vi "Grid_GetAttributes.vi"(0 "reference in":refnum<class "Grid.lvclass">, 5 "error in (no error)":errorcluster) -> (14 "reference out":refnum<class "Grid.lvclass">, 16 "Attributes":T1 {"gridY" format="%.2f"; "gridX" format="%.2f"}, 17 "Attributes locked?":bool, 19 "error out":errorcluster)   [LabVIEW 2012, in "Grid.lvclass"]
doc: "Returns the attributes of a Grid or subclass object.\n\nIf the object is currently locked for modification, 'Attibutes locked?' will return TRUE.\n\n[GOOP 2.0.15]"
uses:
  <resource>/Framework/Providers/Open_GDS/UML/Grid_class/Grid.lvclass
  <resource>/Framework/Providers/Open_GDS/UML/Grid_class/protected/ObjectAttributes.ctl
  <vilib>/addons/_goop3.llb/3GOOPStates.ctl
  <resource>/Framework/Providers/Open_GDS/UML/Grid_class/Grid.lvclass/Grid.ctl
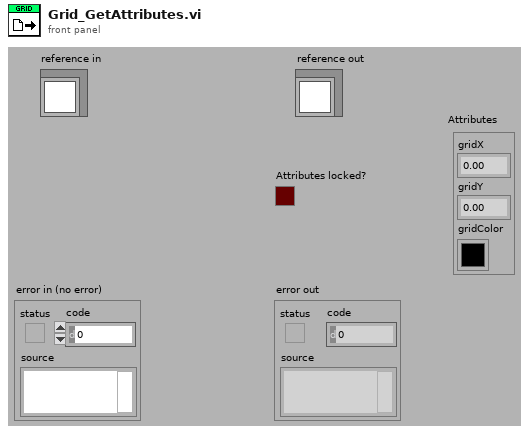
[diagram p1: front panel]
types:
  T1 = typedef "Grid.lvclass/ObjectAttributes.ctl" = cluster{"gridX":dbl, "gridY":dbl, "gridColor":u32}
  T2 = typedef "3GOOPStates.ctl" = enum16{"Set", "Get", "New", "Delete", "Clear", "Test and get", "Unlock data", "Information", "Look up existing", "New or look up existing", "Test and get shared", "Get shared", "Set shared", "Unlock shared", "Find dynamic method", "Register dynamic method", "Preload dynamic method", "Probe", "Cast to more generic", "Cast to more specific"}
  T3 = typedef "Grid.lvclass/ObjectReference.ctl" = refnum<k1>
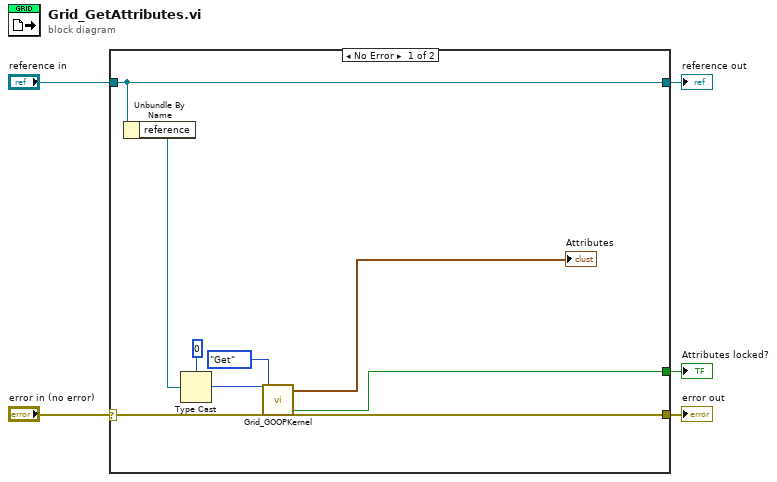
[diagram p0: block diagram]
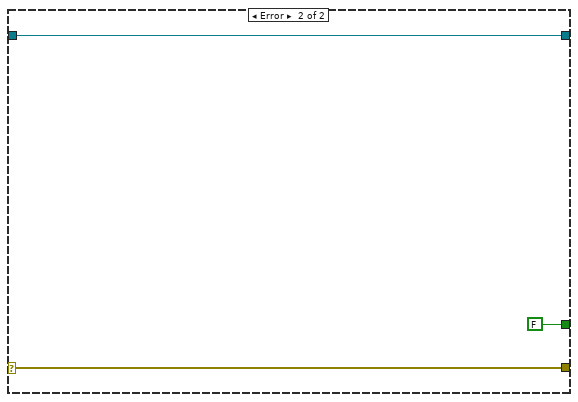
[diagram p2: hidden frame]
diagram:
  n1 = case shown="No Error" "error in (no error)" {
    selector: "error in (no error)" -> [w13 w16]
    tunnel: [w7 w17] -> w5
    tunnel: [w11 w16] -> w4
    tunnel: "reference in" -> [w7 w17]
    tunnel: [w10 FALSE ("Data locked?")] -> w1
    frame No Error {
      n2 = Unbundle By Name(w7) -> ("reference"=w6:T3)
      n3 = Type Cast(type=0, x=w6) -> (*(type *) &x=w12:i32)
      n4 = call <resource>:"Grid_GOOPKernel.vi"("Ref in"=w12, "error in (no error)"=w13, "Action"=3GOOPStates."Get") -> ("Data out"=→"Attributes":T1, "Data locked?"=w10:bool, "error out"=w11:errorcluster)  [unwired: 12 in, 10 out]
    }
    frame Error {
    }
  }
  "error out" <- w4
  "reference out" <- w5
  "Attributes locked?" <- w1
